vi "Generate multi tone waveform.vi"(6 "queue":refnum<queue>, 8 "error in":errorcluster, 9 "Measurement Configuration":T1={"Analog Source Resource Name"="", "IMD Standard"=0, "Custom Low Frequency"=14000.0, "Custom High frequency"=15000.0, "Custom Amplitude Ratio"=1.0, "Amplitude"=-1.0, "Protocol Source Resource Name"="7821\\PCMi 0", "Input range"=2.825, "Number of Words"=19200, "Clock Rate"=12288000, "Latch Delay"=0.0} {"Custom Amplitude Ratio" format="%.1f"; "Custom High frequency" format="%_2p"; "Custom Low Frequency" format="%#_2p"; "Clock Rate" format="%.4p"}, 10 "Sample Rate (Hz)":dbl=51200.0, 11 "task/channels in":refnum<k21>) -> (0 "error out":errorcluster, 3 "task out":refnum<k21>)   [LabVIEW 2021, in "audio_intermodulationDistortionMeasurement.lvlib"]
uses:
  audio_intermodulationDistortionMeasurement.lvlib
  <vilib>/addons/_NISVFA/_Generation/Signal Generation/SV Signal/sv_System Timing Model.ctl
  <vilib>/DAQmx/write.llb/DAQmx Write (Analog 1D Wfm NChan NSamp).vi
  <vilib>/addons/_NISVFA/_Generation/Signal Generation/SV Multitone/SV Multitone.lvclass
  C:/Program Files/National Instruments/LabVIEW 2021/vi.lib/addons/_NISVFA/_Generation/Signal Generation/SV Signal/SV Signal.lvclass
  <vilib>/addons/_NISVFA/_Generation/Signal Generation/SV Signal/Write Sample Rate.vi
  <vilib>/addons/_NISVFA/_Generation/Signal Generation/SV Signal/Write System Timing Model.vi
  <vilib>/addons/_NISVFA/_Generation/Signal Generation/SV Signal/Write Ramp Parameters.vi
  <vilib>/DAQmx/miscellaneous.llb/DAQmx Fill In Error Info.vi
  <vilib>/addons/_NISVFA/_Generation/Signal Generation/SV Multitone/Configure Multitone (Custom).vi
  <vilib>/addons/_NISVFA/_Generation/Signal Generation/SV Signal/SV Signal.lvclass
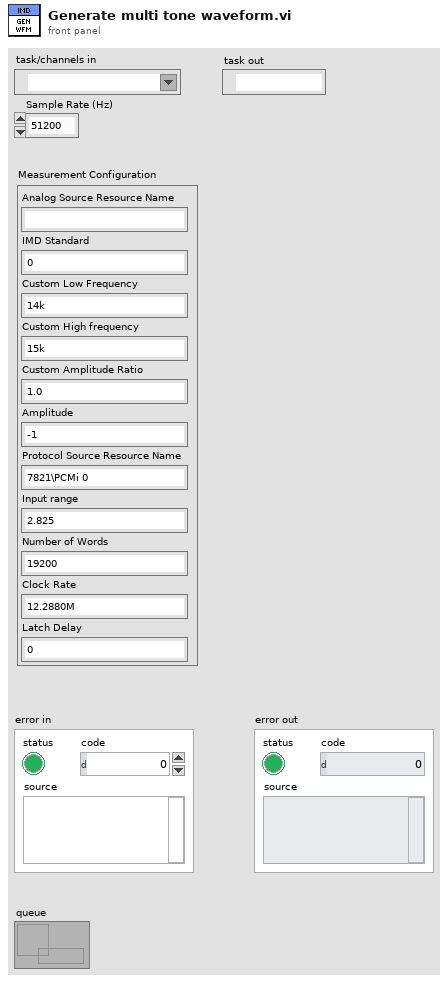
[diagram p1: front panel]
types:
  T1 = cluster{"Analog Source Resource Name":string, "IMD Standard":u16, "Custom Low Frequency":dbl, "Custom High frequency":dbl, "Custom Amplitude Ratio":dbl, "Amplitude":dbl, "Protocol Source Resource Name":string, "Input range":dbl, "Number of Words":i32, "Clock Rate":u32, "Latch Delay":dbl}
  T2 = cluster{"profile":enum16{"Linear", "Half cosine"}, "durations [s]":cluster{"ramp-up":dbl, "transition":dbl, "ramp-down":dbl}}
  T3 = typedef "SV Signal.lvclass/sv_System Timing Model.ctl" = i64
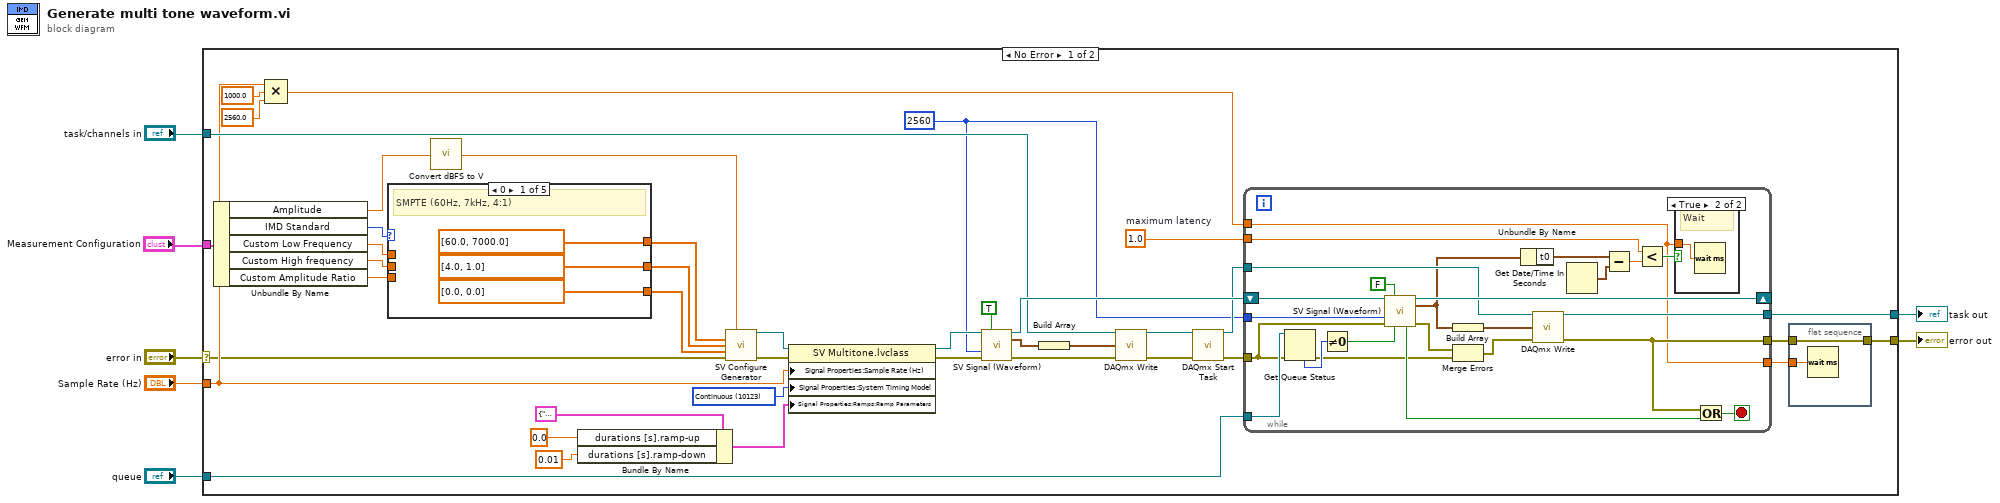
[diagram p0: block diagram]
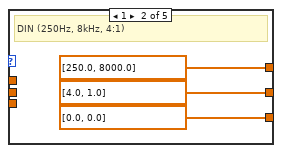
[diagram p3: hidden frame]
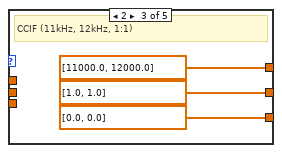
[diagram p4: hidden frame]
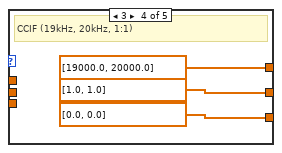
[diagram p5: hidden frame]
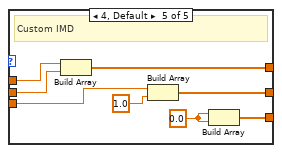
[diagram p6: hidden frame]
diagram:
  n1 = case shown="No Error" "error in" {
    selector: "error in" -> [w8 w97]
    tunnel: [w11 w97] -> w6
    tunnel: "Measurement Configuration" -> [w48 _]
    tunnel: "task/channels in" -> [w25 w96]
    tunnel: "Sample Rate (Hz)" -> [w16 _]
    tunnel: [w10 w96] -> w3
    tunnel: "queue" -> [w9 _]
    frame No Error {
      w18 = 1.0  # maximum latency
      w34 = T3 10123 items=["Finite"=10178, "-"=-1, "Continuous"=10123, "-"=-2, "Settled"=110123, "Averaged"=210123, "Discrete Sweep"=310123, "Continuous Sweep"=410123] ("System Timing Model")
      w19 = 2560 ("samples")
      n2 = Unbundle By Name(w48) -> ("Amplitude"=w43:dbl, "IMD Standard"=w47:u16, "Custom Low Frequency"=w46:dbl, "Custom High frequency"=w45:dbl, "Custom Amplitude Ratio"=w44:dbl)
      n3 = Compound Arithmetic op=MULTIPLY(w16, 1000.0 ("value"), 2560.0 ("value")) -> (w17:dbl)
      n4 = case shown="0" w47 {
        tunnel: [dbl[] [60.0, 7000.0] ("source settings.frequencies") dbl[] [250.0, 8000.0] ("source settings.frequencies") dbl[] [11000.0, 12000.0] ("source settings.frequencies") dbl[] [19000.0, 20000.0] ("source settings.frequencies") w93] -> w42
        tunnel: [dbl[] [4.0, 1.0] ("source settings.frequencies") dbl[] [4.0, 1.0] ("source settings.frequencies") dbl[] [1.0, 1.0] ("source settings.frequencies") dbl[] [1.0, 1.0] ("source settings.frequencies") w92] -> w41
        tunnel: [dbl[] [0.0, 0.0] ("source settings.frequencies") dbl[] [0.0, 0.0] ("source settings.frequencies") dbl[] [0.0, 0.0] ("source settings.frequencies") dbl[] [0.0, 0.0] ("source settings.frequencies") w91] -> w40
        tunnel: w46 -> [_ _ _ _ w90]
        tunnel: w45 -> [_ _ _ _ w89]
        tunnel: w44 -> [_ _ _ _ w88]
        frame 0 {
          # "SMPTE (60Hz, 7kHz, 4:1)"
        }
        frame 1 {
          # "DIN (250Hz, 8kHz, 4:1)"
        }
        frame 2 {
          # "CCIF (11kHz, 12kHz, 1:1)"
        }
        frame 3 {
          # "CCIF (19kHz, 20kHz, 1:1)"
        }
        frame 4, Default {
          w94 = 0.0 ("element")
          # "Custom IMD"
          n5 = Build Array(w90, w89) -> (w93:dbl[])
          n6 = Build Array(w88, 1.0 ("element")) -> (w92:dbl[])
          n7 = Build Array(w94, w94) -> (w91:dbl[])
        }
      }
      n8 = call "Convert dBFS to V.vi"("Amplitude (dBFS)"=w43) -> ("Amplitude (V)"=w39:dbl)
      n9 = Bundle By Name(cluster=T2 {"profile"=enum."Linear", "durations [s]"={"ramp-up"=0.0, "transition"=0.0, "ramp-down"=0.0}} ("Ramp Parameters:All Elements"), "durations [s].ramp-up"=0.0, "durations [s].ramp-down"=0.01) -> (w32:T2)
      n10 = call-poly <vilib>:"SV Configure Generator.vi"("overall amplitude"=w39, "frequencies [Hz]"=w42, "amplitudes"=w41, "phases [deg]"=w40, "error in (no error)"=w8) -> ("signal configuration"=w38:refnum<class "SV Multitone.lvclass">, "error out"=w36:errorcluster)  [unwired: 8 in, 1 out]
      n11 = property class="SV Multitone.lvclass"(reference=w38, error in=w36, "Signal Properties:Sample Rate (Hz)"=w16, "Signal Properties:System Timing Model"=w34, "Signal Properties:Ramps:Ramp Parameters"=w32) -> (reference out=w37:refnum<class "SV Multitone.lvclass">, error out=w35:errorcluster)
      n12 = call-dynamic "SV Signal (Waveform).vi"("signal configuration"=w37, "reset"=TRUE, "samples"=w19, "error in (no error)"=w35) -> ("signal configuration"=w28:refnum<class "SV Multitone.lvclass">, "output waveform"=w29:waveform(dbl), "error out"=w21:errorcluster)  [unwired: 6 in, 3 out]
      n13 = Build Array(w29) -> (w27:waveform(dbl)[])
      n14 = call-poly <vilib>:"DAQmx Write.vi"("task/channels in"=w25, "data"=w27, "error in"=w21) -> ("task out"=w26:refnum<k21>, "error out"=w22:errorcluster)  [unwired: 10 in, 1 out]
      n15 = call <vilib>:"DAQmx Start Task.vi"("task/channels in"=w26, "error in"=w22) -> ("task out"=w23:refnum<k21>, "error out"=w20:errorcluster)  [unwired: 12 in]
      n16 = while {
        shift-right: [w73] -> _
        shift-left: w28 -> [w74]
        tunnel: w19 -> [w62]
        tunnel: w23 -> [w70]
        tunnel: [w69] -> w10
        tunnel: [w68] -> w12
        tunnel: w18 -> [w64]
        tunnel: w17 -> [w59]
        tunnel: [w59] -> w13
        tunnel: w20 -> [w54]
        tunnel: w9 -> [w55]
        stop <- w72 stop-if-true
        n17 = Get Queue Status(queue=w55, error in (no error)=w54) -> (error out=w51:errorcluster, # elements in queue=w57:i32)  [unwired: 1 in, 6 out]
        n18 = Not Equal To 0?(x=w57) -> (x != 0?=w56:bool)
        n19 = call-dynamic "SV Signal (Waveform).vi"("signal configuration"=w74, "reset"=FALSE, "samples"=w62, "error in (no error)"=w54, "stop"=w56) -> ("signal configuration"=w73:refnum<class "SV Multitone.lvclass">, "output waveform"=w61:waveform(dbl), "done"=w71:bool, "error out"=w53:errorcluster)  [unwired: 5 in, 2 out]
        n20 = Build Array(w61) -> (w60:waveform(dbl)[])
        n21 = Merge Errors(w53, w51) -> (w52:errorcluster)
        n22 = Unbundle By Name(w61) -> ("t0"=w67:timestamp)
        n23 = call-poly <vilib>:"DAQmx Write.vi"("task/channels in"=w70, "data"=w60, "error in"=w52) -> ("task out"=w69:refnum<k21>, "error out"=w68:errorcluster)  [unwired: 10 in, 1 out]
        n24 = Get Date/Time In Seconds() -> (seconds since 1Jan1904=w66:timestamp)
        n25 = Subtract(x=w67, y=w66) -> (x-y=w65:dbl)
        n26 = Less?(x=w64, y=w65) -> (x < y?=w63:bool)
        n27 = case shown="True" w63 {
          tunnel: w59 -> [_ w75]
          frame False {
          }
          frame True {
            # "Wait"
            n28 = Wait (ms)(milliseconds to wait=w75) -> ()  [unwired: 1 out]
          }
        }
        n29 = Or(x=w68, y=w71) -> (x .or. y?=w72:bool)
      }
      n30 = flat-sequence {
        tunnel: w13 -> [w50]
        tunnel: w12 -> [w49]
        tunnel: [w49] -> w11
        frame #0 {
          n31 = Wait (ms)(milliseconds to wait=w50) -> ()  [unwired: 1 out]
        }
      }
    }
    frame Error {
    }
  }
  "error out" <- w6
  "task out" <- w3
